vi "set_zone_properties.vi"() -> ()   [LabVIEW 2016]
uses:
  Instrument_Setup.vi
panel:
  in  "Pfad zu HeaterTable":path=path "D:/Cryostat Software/CryoTUM-V1.0/sub_vi-s/Heater Tables/HeaterTableLS370.txt"
  out "HeaterZone Tuning Table.txt":string caption="PID Table"
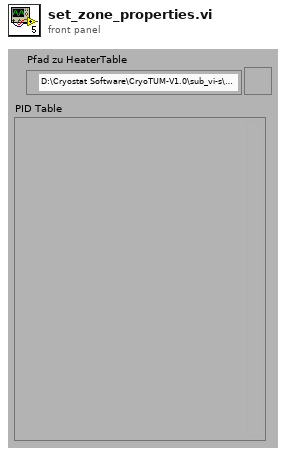
[diagram p1: front panel]
types:
  T1 = enum16{"open", "replace", "create", "open or create", "replace or create", "replace or create with confirmation"}
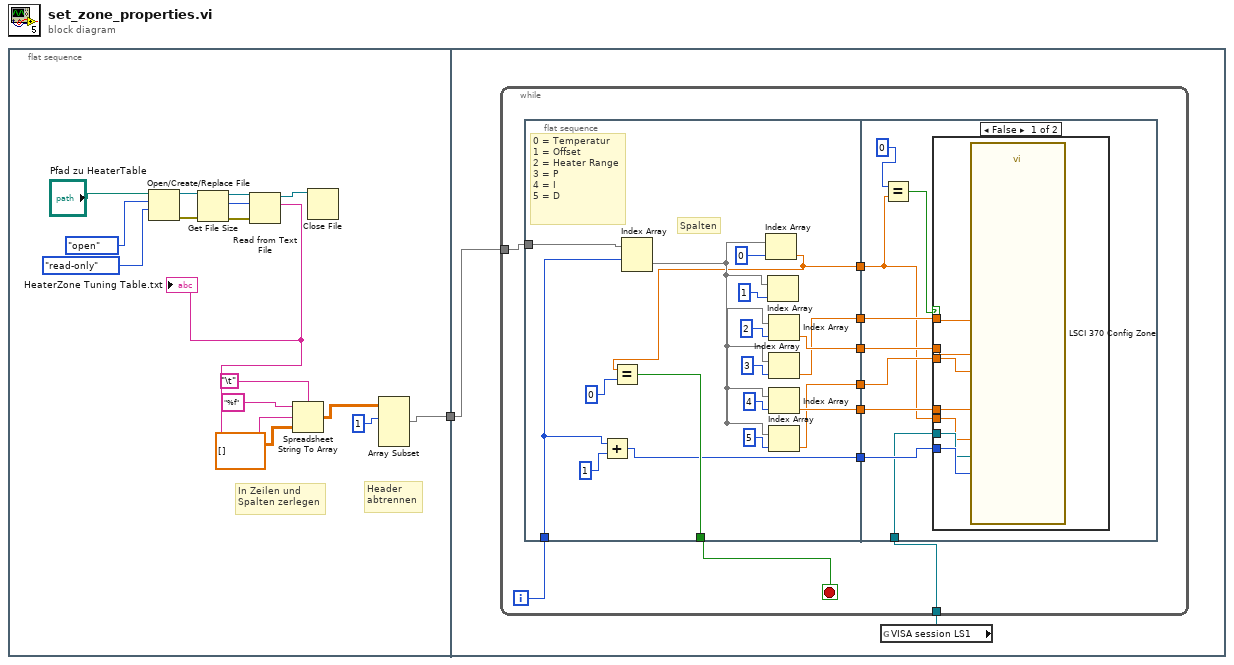
[diagram p0: block diagram]
diagram:
  n1 = flat-sequence {
    tunnel: [w2] -> w1
    tunnel: w1 -> [w19]
    frame #0 {
      # "In Zeilen und \nSpalten zerlegen"
      # "Header\nabtrennen"
      n2 = Open/Create/Replace File(file path (use dialog)="Pfad zu HeaterTable", operation (0:open)=T1."open", access (0:read/write)=enum16{"read/write", "read-only", "write-only"}."read-only") -> (refnum out=w12:refnum<file>, error out=w14:errorcluster)  [unwired: 3 in, 1 out]
      n3 = Get File Size(file=w12, error in=w14) -> (refnum out=w11:refnum<file>, size (in bytes)=w7:i64, 0:w13:errorcluster)
      n4 = Read from Text File(file (use dialog)=w11, count=w7, error in=w13) -> (refnum out=w10:refnum<file>, text=w6:string)  [unwired: 1 in, 2 out]
      "HeaterZone Tuning Table.txt" <- w6
      n5 = Spreadsheet String To Array ("Tabellen-String nach Array")(delimiter (Tab)="\t", format string="%f", spreadsheet string=w6, array type (2D Dbl)=dbl[][] []) -> (array=w5:dbl[][])
      n6 = Close File(refnum=w10) -> ()  [unwired: 1 in, 2 out]
      n7 = Array Subset(array=w5, index (row)=1) -> (w2:dbl[][])  [unwired: 3 in]
    }
    frame #1 {
      n8 = global read "Instrument_Setup.vi" "VISA session LS1"() -> (w18:refnum<visa-resource-name>)
      n9 = while {
        tunnel: w19 -> [w28]
        tunnel: w18 -> [w25]
        i -> [w29]
        stop <- w27 stop-if-true
        n10 = flat-sequence {
          tunnel: w28 -> [w40]
          tunnel: w29 -> [w36]
          tunnel: [w38] -> w27
          tunnel: [w35] -> w26
          tunnel: [w34] -> w24
          tunnel: [w33] -> w23
          tunnel: [w32] -> w22
          tunnel: [w31] -> w21
          tunnel: [w30] -> w20
          tunnel: w26 -> [w56]
          tunnel: w25 -> [w55]
          tunnel: w24 -> [w50]
          tunnel: w23 -> [w54]
          tunnel: w22 -> [w53]
          tunnel: w21 -> [w52]
          tunnel: w20 -> [w51]
          frame #0 {
            # "0 = Temperatur\n1 = Offset\n2 = Heater Range\n3 = P\n4 = I\n5 = D"
            # "Spalten"
            n11 = Add(x=w36, y=1) -> (x+y=w35:i32)
            n12 = Index Array(array=w40, index (row)=w36) -> (element=w42:dbl[])  [unwired: 1 in]
            n13 = Index Array(array=w42, index=0) -> (element=w34:dbl)
            n14 = Equal?(x=w34, y=0) -> (x = y?=w38:bool)
            n15 = Index Array(array=w42, index=1) -> ()  [unwired: 1 out]
            n16 = Index Array(array=w42, index=2) -> (element=w33:dbl)
            n17 = Index Array(array=w42, index=3) -> (element=w32:dbl)
            n18 = Index Array(array=w42, index=4) -> (element=w31:dbl)
            n19 = Index Array(array=w42, index=5) -> (element=w30:dbl)
          }
          frame #1 {
            n20 = Equal?(x=0, y=w50) -> (x = y?=w48:bool)
            n21 = case shown="False" w48 {
              tunnel: w56 -> [w63 _]
              tunnel: w55 -> [w62 _]
              tunnel: w50 -> [w61 _]
              tunnel: w54 -> [w60 _]
              tunnel: w53 -> [w59 _]
              tunnel: w52 -> [w58 _]
              tunnel: w51 -> [w57 _]
              frame False {
                n22 = call "LSCI 370 Config Zone.vi"("VISA session"=w62, "Zone (1)"=w63, "Setpoint Limit (0.00000E+0)"=w61, "Heater Range (0: Off)"=w60, "Gain (P) (10.000)"=w59, "Reset (I) (20)"=w58, "Rate (D) (0)"=w57) -> ()  [unwired: 19 in, 2 out]
              }
              frame True {
              }
            }
          }
        }
      }
    }
  }
